vi "Set_Focus_Plane.vi"(10 "Image Acquisition Parameters Out":T1 {"Z Steps Size (um)" min=0.0; "Number of Z Steps" min=1; "Frames Accumulations" min=1; "Frames Per Capture" min=1; "Line Accumulations" min=1; "Image Format" items=["64 x 64"=64, "128 x 128"=128, "256 x 256"=256, "512 x 512"=512, "1024 x 1024"=1024, "2048 x 2048"=2048]}, 11 "IntensityGraph in":refnum<vi>) -> ()   [LabVIEW 2016]
uses:
  Type Defs/Image Acquisition Parameters.ctl
panel:
  # "Copyright (C) 2020 Edward S Allgeyer\n\nRedistribution and use in source and binary forms, with or without\nmodification, are permitted provided that the following conditions\nare met:\n\n1. Redistributions of source code must retain the above copyright\n   notice, this list of conditions and the following disclaimer.\n\n2. Redistributions in binary form must reproduce the above copyright\n   notice, this list of conditions and the following disclaimer in\n   the documentation and/or other materials provided with the\n   distribution.\n\n3. Neither the name of the copyright holder nor the names of its\n   contributors may be used to endorse or promote products derived\n   from this software without specific prior written permission.\n\nTHIS SOFTWARE IS PROVIDED BY THE COPYRIGHT HOLDERS AND CONTRIBUTORS\n\"AS IS\" AND ANY EXPRESS OR IMPLIED WARRANTIES, INCLUDING, BUT NOT\nLIMITED TO, THE IMPLIED WARRANTIES OF MERCHANTABILITY AND FITNESS\nFOR A PARTICULAR PURPOSE ARE DISCLAIMED. IN NO EVENT SHALL THE\nCOPYRIGHT HOLDER OR CONTRIBUTORS BE LIABLE FOR ANY DIRECT, INDIRECT,\nINCIDENTAL, SPECIAL, EXEMPLARY, OR CONSEQUENTIAL DAMAGES (INCLUDING,\nBUT NOT LIMITED TO, PROCUREMENT OF SUBSTITUTE GOODS OR SERVICES;\nLOSS OF USE, DATA, OR PROFITS; OR BUSINESS INTERRUPTION) HOWEVER\nCAUSED AND ON ANY THEORY OF LIABILITY, WHETHER IN CONTRACT, STRICT\nLIABILITY, OR TORT (INCLUDING NEGLIGENCE OR OTHERWISE) ARISING IN\nANY WAY OUT OF THE USE OF THIS SOFTWARE, EVEN IF ADVISED OF THE\nPOSSIBILITY OF SUCH DAMAGE."
  # "XY"
  # "Z"
  # "Length"
  # "Height"
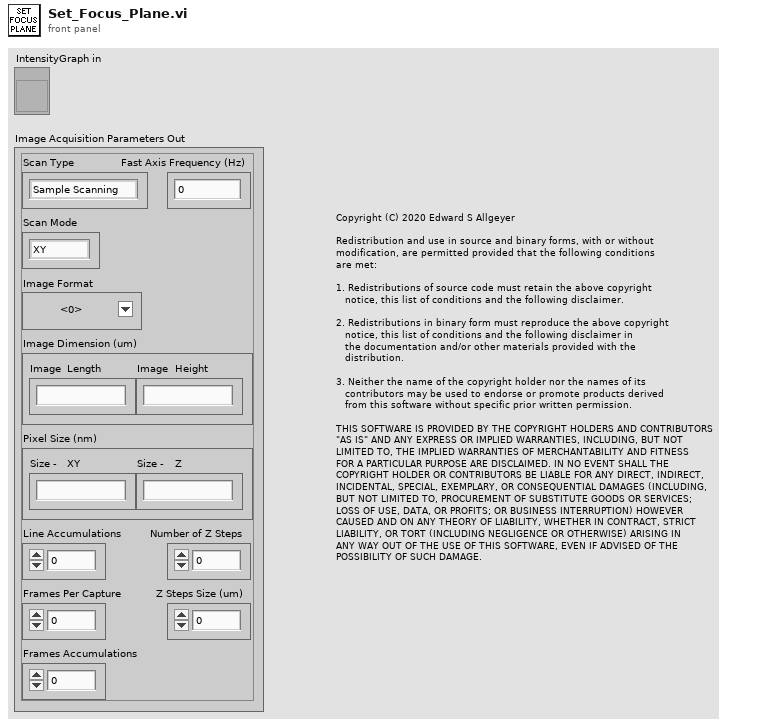
[diagram p1: front panel]
types:
  T1 = typedef "Image Acquisition Parameters.ctl" = cluster{"Scan Type":enum16{"Sample Scanning", "Beam Scanning"}, "Scan Mode":enum16{"XY", "XZ", "YZ", "XYZ"}, "Fast Axis Frequency (Hz)":dbl, "Image Format":u16, "Line Accumulations":u16, "Frames Per Capture":u16, "Frames Accumulations":u16, "Image Dimension (um)":dbl[], "Number of Z Steps":u8, "Z Steps Size (um)":dbl, "Pixel Size (nm)":dbl[]}
  T2 = typedef "Scanning Conversions.ctl" = cluster{"Stage X Axis (Volts/um)":dbl, "Stage Y Axis (Volts/um)":dbl, "Stage Z Axis (Volts/um)":dbl}
  T3 = typedef "Scan Parameters.ctl" = cluster{"Fast_Ax_Amp_V":dbl, "Fast_Ax_Off_V":dbl, "Slow_Ax_Amp_V":dbl, "Slow_Ax_Off_V ":dbl, "Slow_Ax_Max_V_VperS":dbl, "Slow_Ax1_Del25ns":i32, "Slow_Ax2_Del25ns":i32, "Stage_X_Off_V":dbl, "Stage_Y_Off_V":dbl, "Stage_Z_Off_V":dbl, "Galvo1_Off_V":dbl, "Galvo2_Off_V":dbl, "Last_Scan_Mode":enum16{"XY", "XZ", "YZ", "XYZ"}, "Current_Scan_Mode":enum16{"XY", "XZ", "YZ", "XYZ"}, "Fly_Back_Lines":u16, "Linear_Ramp_End":u32, "Z_Step_I16":i16, "Z_Start_I16":i16, "Laser_States _U32":u32, "590_Voltage_I16":i16, "775_AOM_Volt_I16":i16, "Blanking OFF":bool, "Unused_Axis_I16":i16}
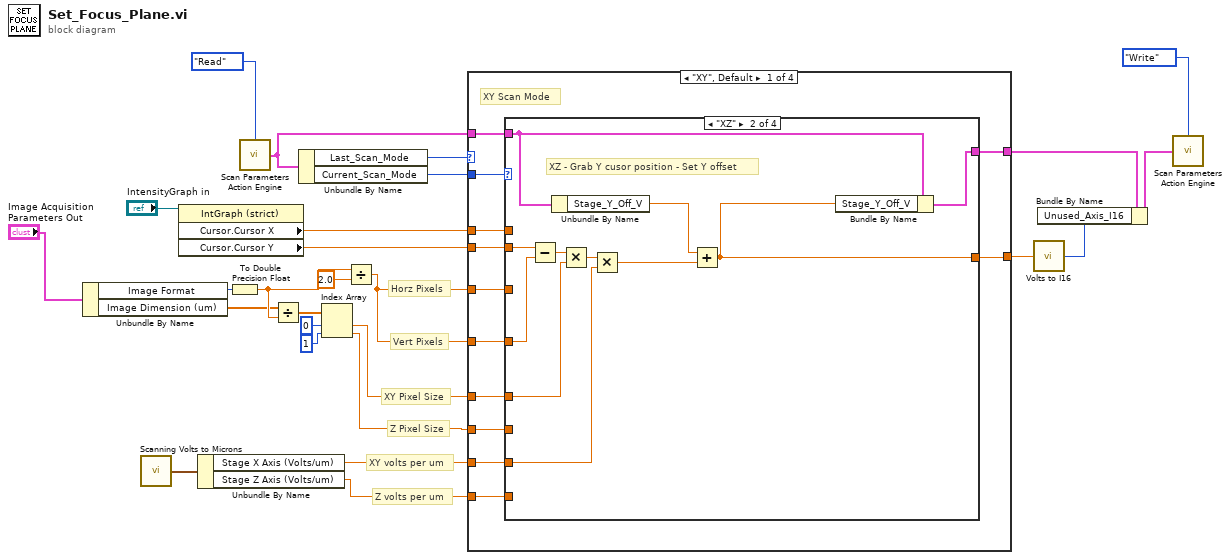
[diagram p0: block diagram]
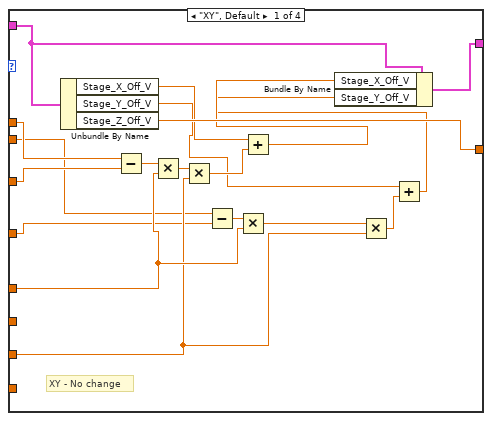
[diagram p2: hidden frame]
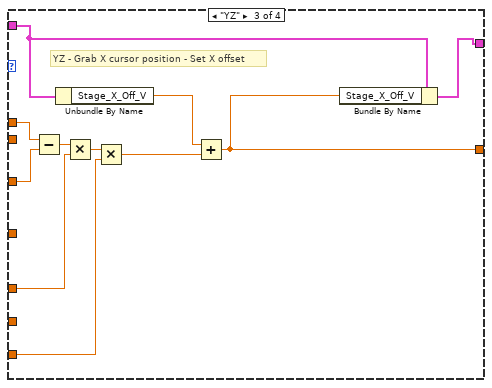
[diagram p3: hidden frame]
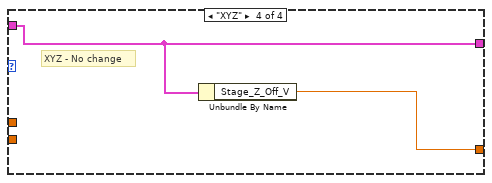
[diagram p4: hidden frame]
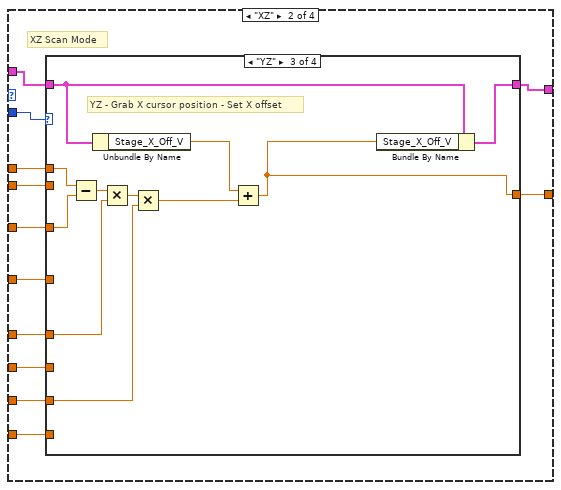
[diagram p5: hidden frame]
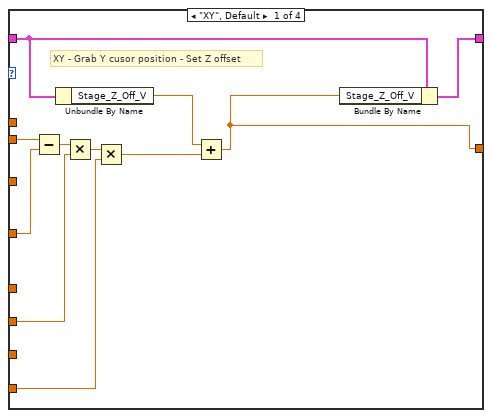
[diagram p6: hidden frame]
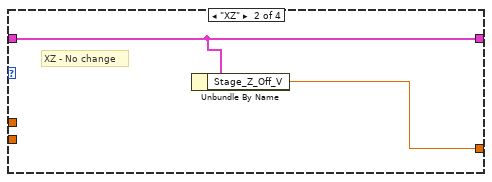
[diagram p7: hidden frame]
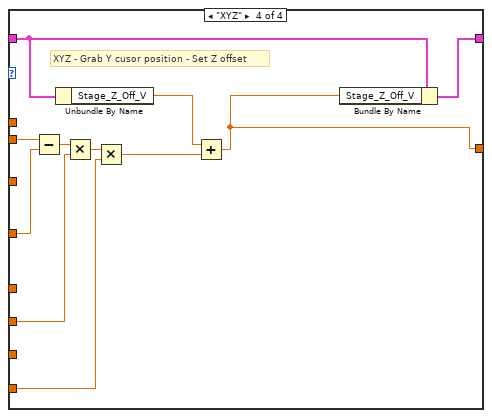
[diagram p8: hidden frame]
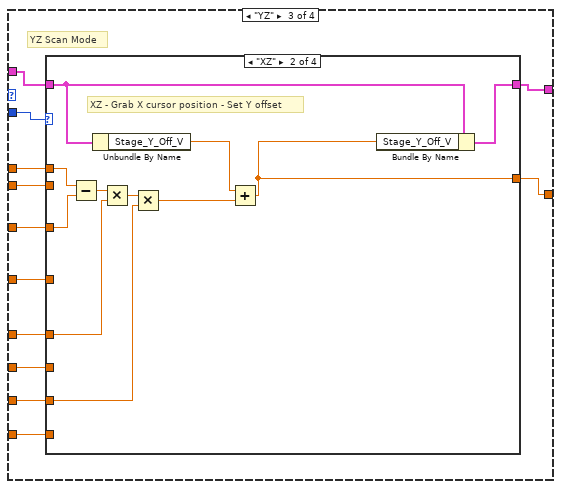
[diagram p9: hidden frame]
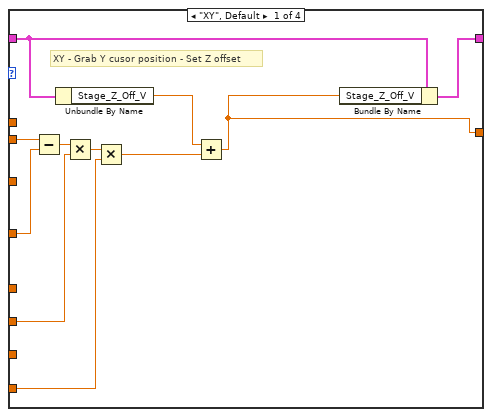
[diagram p10: hidden frame]
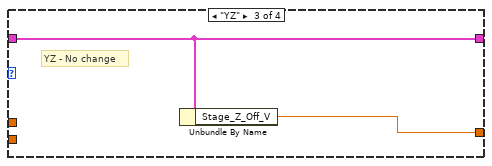
[diagram p11: hidden frame]
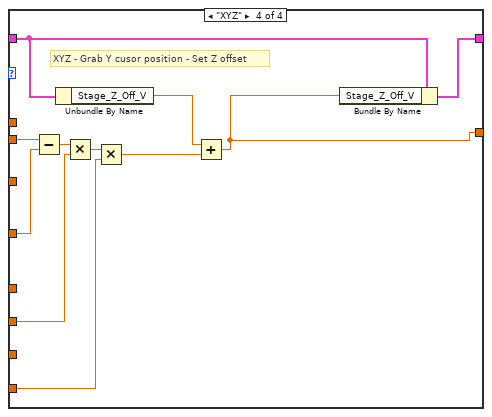
[diagram p12: hidden frame]
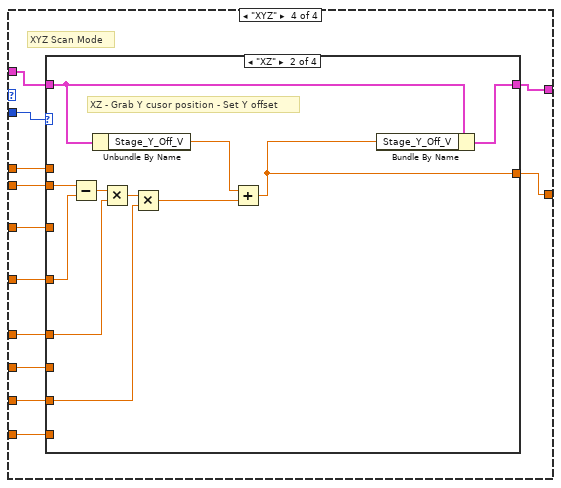
[diagram p13: hidden frame]
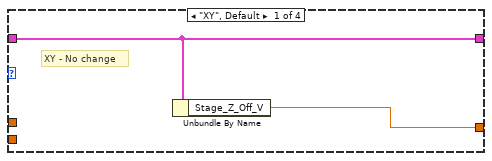
[diagram p14: hidden frame]
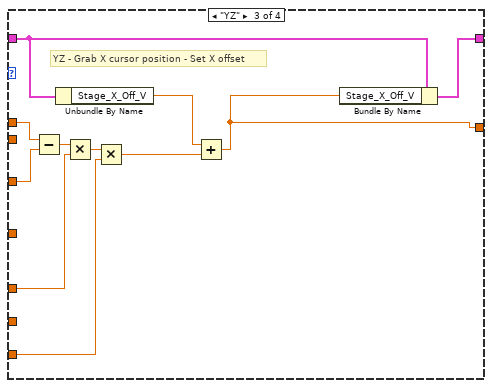
[diagram p15: hidden frame]
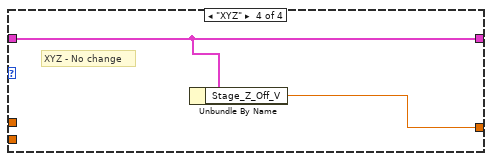
[diagram p16: hidden frame]
diagram:
  # "Vert Pixels"
  # "Horz Pixels"
  # "Z Pixel Size"
  # "XY Pixel Size"
  # "Z volts per um"
  # "XY volts per um"
  n1 = Unbundle By Name("Image Acquisition Parameters Out") -> ("Image Format"=w11:u16, "Image Dimension (um)"=w8:dbl[])
  n2 = call "Scanning Volts to Microns.vi"() -> ("Scanning Conversions OUT"=w21:T2)
  n3 = property on="Property Node" class="IntGraph (strict)"(reference="IntensityGraph in") -> ("Cursor.Cursor X"=w16:dbl, "Cursor.Cursor Y"=w15:dbl)  [unwired: 1 in, 2 out]
  n4 = Unbundle By Name(w21) -> ("Stage X Axis (Volts/um)"=w22:dbl, "Stage Z Axis (Volts/um)"=w23:dbl)
  n5 = To Double Precision Float(number=w11) -> (double precision float=w18:dbl)
  n6 = call "Scan Parameters Action Engine.vi"("Action"=enum16{"Read", "Write"}."Read") -> ("Scan Parameters OUT"=w3:T3)  [unwired: 14 in]
  n7 = Divide(x=w8, y=w18) -> (x/y=w7:dbl[])
  n8 = Unbundle By Name(w3) -> ("Last_Scan_Mode"=w13:enum16{"XY", "XZ", "YZ", "XYZ"}, "Current_Scan_Mode"=w12:enum16{"XY", "XZ", "YZ", "XYZ"})
  n9 = Index Array(array=w7, index #1=0 ("index"), index #2=1 ("index")) -> (element #1=w6:dbl, element #2=w5:dbl)
  n10 = Divide(x=w18, y=2.0) -> (x/y=w19:dbl)
  n11 = case shown="\"XY\", Default" w13 {
    tunnel: w12 -> [w30 w93 w140 w187]
    tunnel: w16 -> [w31 w85 w132 w179]
    tunnel: w15 -> [w32 w86 w133 w180]
    tunnel: w19 -> [w38 w92 w139 w186]
    tunnel: w6 -> [w37 w91 w138 w185]
    tunnel: w23 -> [w35 w89 w136 w183]
    tunnel: w22 -> [w36 w90 w137 w184]
    tunnel: w5 -> [w34 w88 w135 w182]
    tunnel: w19 -> [w33 w87 w134 w181]
    tunnel: w3 -> [w29 w84 w131 w178]
    tunnel: [w28 w83 w130 w177] -> w24
    tunnel: [w27 w82 w129 w176] -> w17
    frame "XY", Default {
      # "XY Scan Mode"
      n12 = case shown="\"XZ\"" w30 {
        tunnel: w38 -> [w47 _ w73 _]
        tunnel: w37 -> [w49 w67 w78 _]
        tunnel: w36 -> [w48 w65 w76 _]
        tunnel: w35 -> [_ _ _ _]
        tunnel: w34 -> [_ _ _ _]
        tunnel: w33 -> [w45 w63 _ _]
        tunnel: w32 -> [w46 w62 _ _]
        tunnel: w31 -> [w54 _ w72 _]
        tunnel: w29 -> [w53 w59 w71 w81]
        tunnel: [w52 w60 w70 w81] -> w28
        tunnel: [w57 w58 w69 w80] -> w27
        frame "XY", Default {
          # "XY - No change"
          n13 = Unbundle By Name(w53) -> ("Stage_X_Off_V"=w43:dbl, "Stage_Y_Off_V"=w41:dbl, "Stage_Z_Off_V"=w57:dbl)
          n14 = Subtract(x=w54, y=w47) -> (x-y=w56:dbl)
          n15 = Multiply(x=w56, y=w49) -> (x*y=w55:dbl)
          n16 = Multiply(x=w55, y=w48) -> (x*y=w44:dbl)
          n17 = Subtract(x=w46, y=w45) -> (x-y=w50:dbl)
          n18 = Multiply(x=w50, y=w49) -> (x*y=w51:dbl)
          n19 = Add(x=w43, y=w44) -> (x+y=w42:dbl)
          n20 = Multiply(x=w51, y=w48) -> (x*y=w40:dbl)
          n21 = Add(x=w41, y=w40) -> (x+y=w39:dbl)
          n22 = Bundle By Name(cluster=w53, "Stage_X_Off_V"=w42, "Stage_Y_Off_V"=w39) -> (w52:T3)
        }
        frame "XZ" {
          # "XZ - Grab Y cusor position - Set Y offset"
          n23 = Subtract(x=w62, y=w63) -> (x-y=w68:dbl)
          n24 = Unbundle By Name(w59) -> ("Stage_Y_Off_V"=w61:dbl)
          n25 = Multiply(x=w68, y=w67) -> (x*y=w66:dbl)
          n26 = Multiply(x=w66, y=w65) -> (x*y=w64:dbl)
          n27 = Add(x=w61, y=w64) -> (x+y=w58:dbl)
          n28 = Bundle By Name(cluster=w59, "Stage_Y_Off_V"=w58) -> (w60:T3)
        }
        frame "YZ" {
          # "YZ - Grab X cursor position - Set X offset"
          n29 = Subtract(x=w72, y=w73) -> (x-y=w79:dbl)
          n30 = Unbundle By Name(w71) -> ("Stage_X_Off_V"=w75:dbl)
          n31 = Multiply(x=w79, y=w78) -> (x*y=w77:dbl)
          n32 = Multiply(x=w77, y=w76) -> (x*y=w74:dbl)
          n33 = Add(x=w75, y=w74) -> (x+y=w69:dbl)
          n34 = Bundle By Name(cluster=w71, "Stage_X_Off_V"=w69) -> (w70:T3)
        }
        frame "XYZ" {
          # "XYZ - No change"
          n35 = Unbundle By Name(w81) -> ("Stage_Z_Off_V"=w80:dbl)
        }
      }
    }
    frame "XZ" {
      # "XZ Scan Mode"
      n36 = case shown="\"YZ\"" w93 {
        tunnel: w92 -> [_ _ w109 _]
        tunnel: w91 -> [_ _ w116 _]
        tunnel: w90 -> [_ _ w113 _]
        tunnel: w89 -> [w96 _ _ w120]
        tunnel: w84 -> [w103 w106 w115 w127]
        tunnel: w88 -> [w95 _ _ w119]
        tunnel: [w100 w106 w110 w124] -> w83
        tunnel: w87 -> [w99 _ _ w123]
        tunnel: w86 -> [w98 _ _ w122]
        tunnel: w85 -> [_ _ w108 _]
        tunnel: [w94 w105 w107 w118] -> w82
        frame "XY", Default {
          # "XY - Grab Y cusor position - Set Z offset"
          n37 = Subtract(x=w98, y=w99) -> (x-y=w104:dbl)
          n38 = Unbundle By Name(w103) -> ("Stage_Z_Off_V"=w97:dbl)
          n39 = Multiply(x=w104, y=w95) -> (x*y=w102:dbl)
          n40 = Multiply(x=w102, y=w96) -> (x*y=w101:dbl)
          n41 = Add(x=w97, y=w101) -> (x+y=w94:dbl)
          n42 = Bundle By Name(cluster=w103, "Stage_Z_Off_V"=w94) -> (w100:T3)
        }
        frame "XZ" {
          # "XZ - No change"
          n43 = Unbundle By Name(w106) -> ("Stage_Z_Off_V"=w105:dbl)
        }
        frame "YZ" {
          # "YZ - Grab X cursor position - Set X offset"
          n44 = Subtract(x=w108, y=w109) -> (x-y=w117:dbl)
          n45 = Unbundle By Name(w115) -> ("Stage_X_Off_V"=w112:dbl)
          n46 = Multiply(x=w117, y=w116) -> (x*y=w114:dbl)
          n47 = Multiply(x=w114, y=w113) -> (x*y=w111:dbl)
          n48 = Add(x=w112, y=w111) -> (x+y=w107:dbl)
          n49 = Bundle By Name(cluster=w115, "Stage_X_Off_V"=w107) -> (w110:T3)
        }
        frame "XYZ" {
          # "XYZ - Grab Y cusor position - Set Z offset"
          n50 = Subtract(x=w122, y=w123) -> (x-y=w128:dbl)
          n51 = Unbundle By Name(w127) -> ("Stage_Z_Off_V"=w121:dbl)
          n52 = Multiply(x=w128, y=w119) -> (x*y=w126:dbl)
          n53 = Multiply(x=w126, y=w120) -> (x*y=w125:dbl)
          n54 = Add(x=w121, y=w125) -> (x+y=w118:dbl)
          n55 = Bundle By Name(cluster=w127, "Stage_Z_Off_V"=w118) -> (w124:T3)
        }
      }
    }
    frame "YZ" {
      # "YZ Scan Mode"
      n56 = case shown="\"XZ\"" w140 {
        tunnel: w139 -> [_ w154 _ _]
        tunnel: w138 -> [_ w161 _ _]
        tunnel: w137 -> [_ w158 _ _]
        tunnel: w136 -> [w143 _ _ w167]
        tunnel: w131 -> [w150 w160 w164 w174]
        tunnel: w135 -> [w142 _ _ w166]
        tunnel: [w147 w155 w164 w171] -> w130
        tunnel: w134 -> [w146 _ _ w170]
        tunnel: w133 -> [w145 _ _ w169]
        tunnel: w132 -> [_ w153 _ _]
        tunnel: [w141 w152 w163 w165] -> w129
        frame "XY", Default {
          # "XY - Grab Y cusor position - Set Z offset"
          n57 = Subtract(x=w145, y=w146) -> (x-y=w151:dbl)
          n58 = Unbundle By Name(w150) -> ("Stage_Z_Off_V"=w144:dbl)
          n59 = Multiply(x=w151, y=w142) -> (x*y=w149:dbl)
          n60 = Multiply(x=w149, y=w143) -> (x*y=w148:dbl)
          n61 = Add(x=w144, y=w148) -> (x+y=w141:dbl)
          n62 = Bundle By Name(cluster=w150, "Stage_Z_Off_V"=w141) -> (w147:T3)
        }
        frame "XZ" {
          # "XZ - Grab X cursor position - Set Y offset"
          n63 = Subtract(x=w153, y=w154) -> (x-y=w162:dbl)
          n64 = Unbundle By Name(w160) -> ("Stage_Y_Off_V"=w157:dbl)
          n65 = Multiply(x=w162, y=w161) -> (x*y=w159:dbl)
          n66 = Multiply(x=w159, y=w158) -> (x*y=w156:dbl)
          n67 = Add(x=w157, y=w156) -> (x+y=w152:dbl)
          n68 = Bundle By Name(cluster=w160, "Stage_Y_Off_V"=w152) -> (w155:T3)
        }
        frame "YZ" {
          # "YZ - No change"
          n69 = Unbundle By Name(w164) -> ("Stage_Z_Off_V"=w163:dbl)
        }
        frame "XYZ" {
          # "XYZ - Grab Y cusor position - Set Z offset"
          n70 = Subtract(x=w169, y=w170) -> (x-y=w175:dbl)
          n71 = Unbundle By Name(w174) -> ("Stage_Z_Off_V"=w168:dbl)
          n72 = Multiply(x=w175, y=w166) -> (x*y=w173:dbl)
          n73 = Multiply(x=w173, y=w167) -> (x*y=w172:dbl)
          n74 = Add(x=w168, y=w172) -> (x+y=w165:dbl)
          n75 = Bundle By Name(cluster=w174, "Stage_Z_Off_V"=w165) -> (w171:T3)
        }
      }
    }
    frame "XYZ" {
      # "XYZ Scan Mode"
      n76 = case shown="\"XZ\"" w187 {
        tunnel: w186 -> [_ _ w203 _]
        tunnel: w185 -> [_ w199 w210 _]
        tunnel: w184 -> [_ w196 w207 _]
        tunnel: w183 -> [_ _ _ _]
        tunnel: w178 -> [w189 w198 w209 w213]
        tunnel: w182 -> [_ _ _ _]
        tunnel: [w189 w194 w204 w213] -> w177
        tunnel: w181 -> [_ w193 _ _]
        tunnel: w180 -> [_ w192 _ _]
        tunnel: w179 -> [_ _ w202 _]
        tunnel: [w188 w190 w201 w212] -> w176
        frame "XY", Default {
          # "XY - No change"
          n77 = Unbundle By Name(w189) -> ("Stage_Z_Off_V"=w188:dbl)
        }
        frame "XZ" {
          # "XZ - Grab Y cusor position - Set Y offset"
          n78 = Subtract(x=w192, y=w193) -> (x-y=w200:dbl)
          n79 = Unbundle By Name(w198) -> ("Stage_Y_Off_V"=w191:dbl)
          n80 = Multiply(x=w200, y=w199) -> (x*y=w197:dbl)
          n81 = Multiply(x=w197, y=w196) -> (x*y=w195:dbl)
          n82 = Add(x=w191, y=w195) -> (x+y=w190:dbl)
          n83 = Bundle By Name(cluster=w198, "Stage_Y_Off_V"=w190) -> (w194:T3)
        }
        frame "YZ" {
          # "YZ - Grab X cursor position - Set X offset"
          n84 = Subtract(x=w202, y=w203) -> (x-y=w211:dbl)
          n85 = Unbundle By Name(w209) -> ("Stage_X_Off_V"=w206:dbl)
          n86 = Multiply(x=w211, y=w210) -> (x*y=w208:dbl)
          n87 = Multiply(x=w208, y=w207) -> (x*y=w205:dbl)
          n88 = Add(x=w206, y=w205) -> (x+y=w201:dbl)
          n89 = Bundle By Name(cluster=w209, "Stage_X_Off_V"=w201) -> (w204:T3)
        }
        frame "XYZ" {
          # "XYZ - No change"
          n90 = Unbundle By Name(w213) -> ("Stage_Z_Off_V"=w212:dbl)
        }
      }
    }
  }
  n91 = call "Volts to I16.vi"("Voltage (V)"=w17) -> ("I16"=w25:i16)  [unwired: 13 in, 1 out]
  n92 = Bundle By Name(cluster=w24, "Unused_Axis_I16"=w25) -> (w26:T3)
  n93 = call "Scan Parameters Action Engine.vi"("Action"=enum16{"Read", "Write"}."Write", "Scan Parameters IN"=w26) -> ()  [unwired: 13 in, 1 out]
